vi "get_scanners.vi"(8 "error in (no error)":errorcluster, 11 "DL090202ScanHead.lvclass in":refnum<class "ScanHeadDL090202.lvclass">) -> (0 "error out":errorcluster, 2 "scanners":refnum<class "GenericSignalWriter.lvclass">[](array[class]), 3 "DL090202ScanHead.lvclass out":refnum<class "ScanHeadDL090202.lvclass">)   [LabVIEW 2010, in "ScanHeadDL090202.lvclass"]
uses:
  ScanHeadDL090202.lvclass
  SignalWriter/GenericSignalWriter/GenericSignalWriter/GenericSignalWriter.lvclass
  ScanHeadDL090202.lvclass/ScanHeadDL090202.ctl
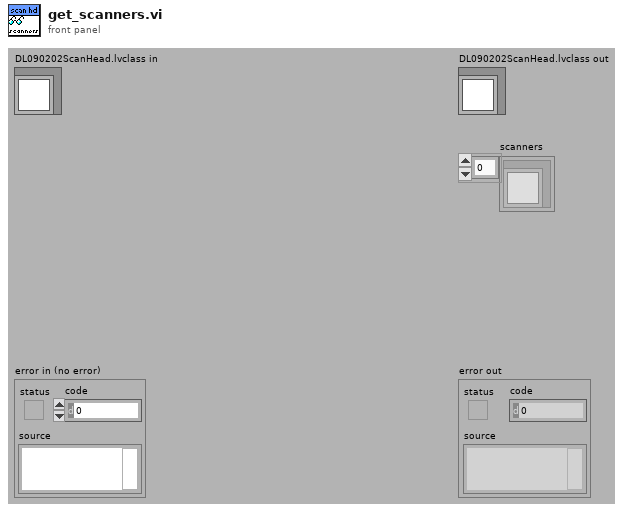
[diagram p1: front panel]
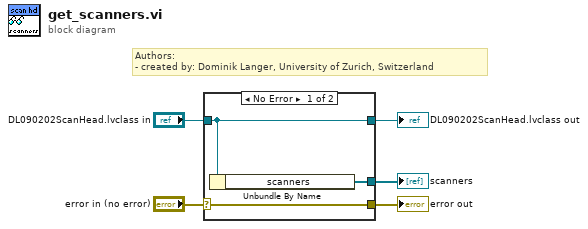
[diagram p0: block diagram]
diagram:
  # "Authors: \n- created by: Dominik Langer, University of Zurich, Switzerland"
  n1 = case shown="No Error" "error in (no error)" {
    selector: "error in (no error)" -> [w8 w9]
    tunnel: [w8 w9] -> w4
    tunnel: [w7 w10] -> w2
    tunnel: "DL090202ScanHead.lvclass in" -> [w7 w10]
    tunnel: [w6 _] -> w1
    frame No Error {
      n2 = Unbundle By Name(w7) -> ("scanners"=w6:refnum<class "GenericSignalWriter.lvclass">[])
    }
    frame Error {
    }
  }
  "error out" <- w4
  "DL090202ScanHead.lvclass out" <- w2
  "scanners" <- w1
